vi "Set defocus array.vi"(8 "error in (no error)":errorcluster, 11 "Autofocus in":refnum<class "Autofocus.lvclass">) -> (0 "error out":errorcluster, 3 "Autofocus out":refnum<class "Autofocus.lvclass">)   [LabVIEW 2012, in "Autofocus.lvclass"]
uses:
  Autofocus.lvclass
  Autofocus.lvclass/Autofocus.ctl
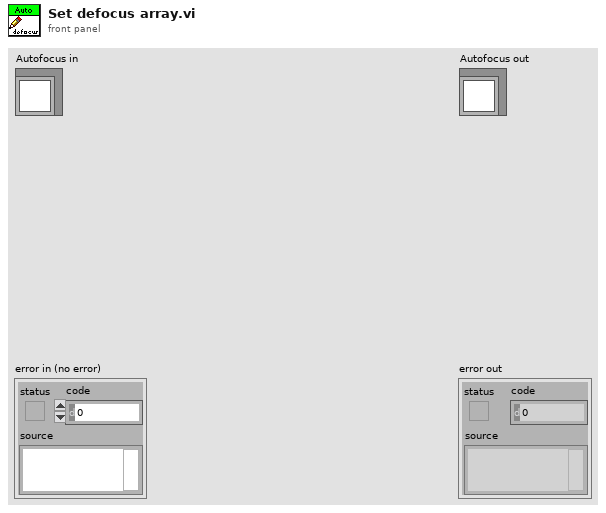
[diagram p1: front panel]
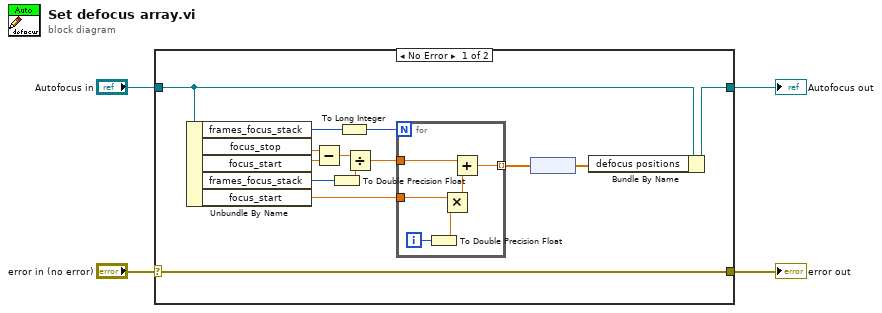
[diagram p0: block diagram]
diagram:
  n1 = case shown="No Error" "error in (no error)" {
    selector: "error in (no error)" -> [w18 w26]
    tunnel: [w18 w26] -> w3
    tunnel: [w7 w25] -> w1
    tunnel: "Autofocus in" -> [w8 w25]
    frame No Error {
      n2 = Unbundle By Name(w8) -> ("frames_focus_stack"=w10:u16, "focus_stop"=w17:dbl[unit], "focus_start"=w16:dbl[unit], "frames_focus_stack"=w14:u16, "focus_start"=w11:dbl[unit])
      n3 = Subtract(x=w17, y=w16) -> (x-y=w15:dbl[unit])
      n4 = To Double Precision Float(number=w14) -> (double precision float=w13:dbl)
      n5 = To Long Integer(number=w10) -> (32bit integer=w9:i32)
      n6 = Divide(x=w15, y=w13) -> (x/y=w12:dbl[unit])
      n7 = for {
        N: w9 -> [_]
        tunnel: w12 -> [w24]
        tunnel: w11 -> [w21]
        tunnel: [w19] -> w6 mode=indexing
        i -> [w23]
        n8 = To Double Precision Float(number=w23) -> (double precision float=w22:dbl)
        n9 = Multiply(x=w21, y=w22) -> (x*y=w20:dbl[unit])
        n10 = Add(x=w24, y=w20) -> (x+y=w19:dbl[unit])
      }
      n11 = node(w6) -> (w5:dbl[])
      n12 = Bundle By Name(cluster=w8, "defocus positions"=w5) -> (w7:refnum<class "Autofocus.lvclass">)
    }
    frame Error {
    }
  }
  "error out" <- w3
  "Autofocus out" <- w1
